vi "引用測試5.vi"() -> ()   [LabVIEW 2015]
uses:
  <vilib>/userdefined/High Color/IMAQdx.ctl
  <vilib>/vision/Measure.llb/Edge Options.ctl
  <vilib>/vision/Measure.llb/Edge Polarity.ctl
  <vilib>/vision/driver/NI_Vision_Acquisition_Software.lvlib
  <vilib>/vision/NI_Vision_Development_Module.lvlib
panel:
  out "error out 2":errorcluster
  in  "Options":T3={"Search Direction"=0, "Edge Options"={"Edge Polarity"=0, "Kernel Size"=3, "Width"=3, "Minimum Edge Strength"=10.0, "Interpolation Type"=enum."Bilinear Fixed", "Data Processing Method"=enum."Average"}, "Show Search Area"=FALSE, "Show Search Lines"=FALSE, "Show Edges Found"=FALSE, "Show Result"=TRUE, "Search Area Color"=65280, "Search Lines Color"=255, "Edge Locations Color"=16776960, "Result Color"=16711680, "Overlay Group Name"=""} {"Edge Options"."Edge Polarity" items=["All Edges", "Rising Edges", "Falling Edges"]; "Edge Options"."Minimum Edge Strength" format="%.2f"; "Edge Options"."Width" step=2; "Edge Options"."Kernel Size" step=2; "Search Direction" items=["Left to Right", "Right to Left", "Top to Bottom", "Bottom to Top"]}
  in  "Tab Control":T4(tab)
  in  "邊":T5(ring)
  out "Line Data":cluster{"X":sgl, "Y":sgl, "T":sgl}
  in  "圓":enum16{"Inner to Outer", "Outer to Inner"}(ring)
  out "Ellipse":T6 {"Minor Axis"."Point 2"."Y" format="%.2f"; "Minor Axis"."Point 2"."X" format="%.2f"; "Minor Axis"."Point 1"."Y" format="%.2f"; "Minor Axis"."Point 1"."X" format="%.2f"; "Major Axis"."Point 2"."Y" format="%.2f"; "Major Axis"."Point 2"."X" format="%.2f"; "Major Axis"."Point 1"."Y" format="%.2f"; "Major Axis"."Point 1"."X" format="%.2f"; "Center"."Y" format="%.2f"; "Center"."X" format="%.2f"}
  in  "線":enum16{"Start to End", "End to Start"}(ring)
  out "Location (Pixel)":cluster{"X":sgl, "Y":sgl}
  in  "DieArea":i32=100 min=10
  in  "ShowData":bool
  in  "抓寬度(方向)":T7(ring)=enum."Horizon(Outer to Inner)"
  in  "Settings":T8={"Contrast"=40, "Filter width"=4, "Steepness"=2, "Subsampling Ratio"=5, "Show Search Area"=FALSE, "Show Search Lines"=FALSE, "Show Edges Found"=FALSE, "Show Result"=TRUE}
  out "Distance":sgl
  in  "繪圖":bool
  in  "繪圖ROI資料":T9=enum."Set Data"
  out "Line Profile":T10(graph)
  in  "Session In":T11="cam1"
  in  "Numeric":i32
  in  "重新開圖":bool
  in  "開圖":bool
  in  "動作":enum16{"什麼也不做", "抓邊", "看灰階", "分析光源均勻度", "抓寬度"}(ring)
  out "Mean":sgl format="%#.2f"
  out "Histogram":T12(graph)
  in  "取像":bool
  out "error out":errorcluster
  out "Gradient Information":dbl[][](graph)
  in  "Process":T13(ring)
  in  "Gap":i32=10 min=1 max=300
  in  "stop":bool
  out "Image":T14(plugin-control)
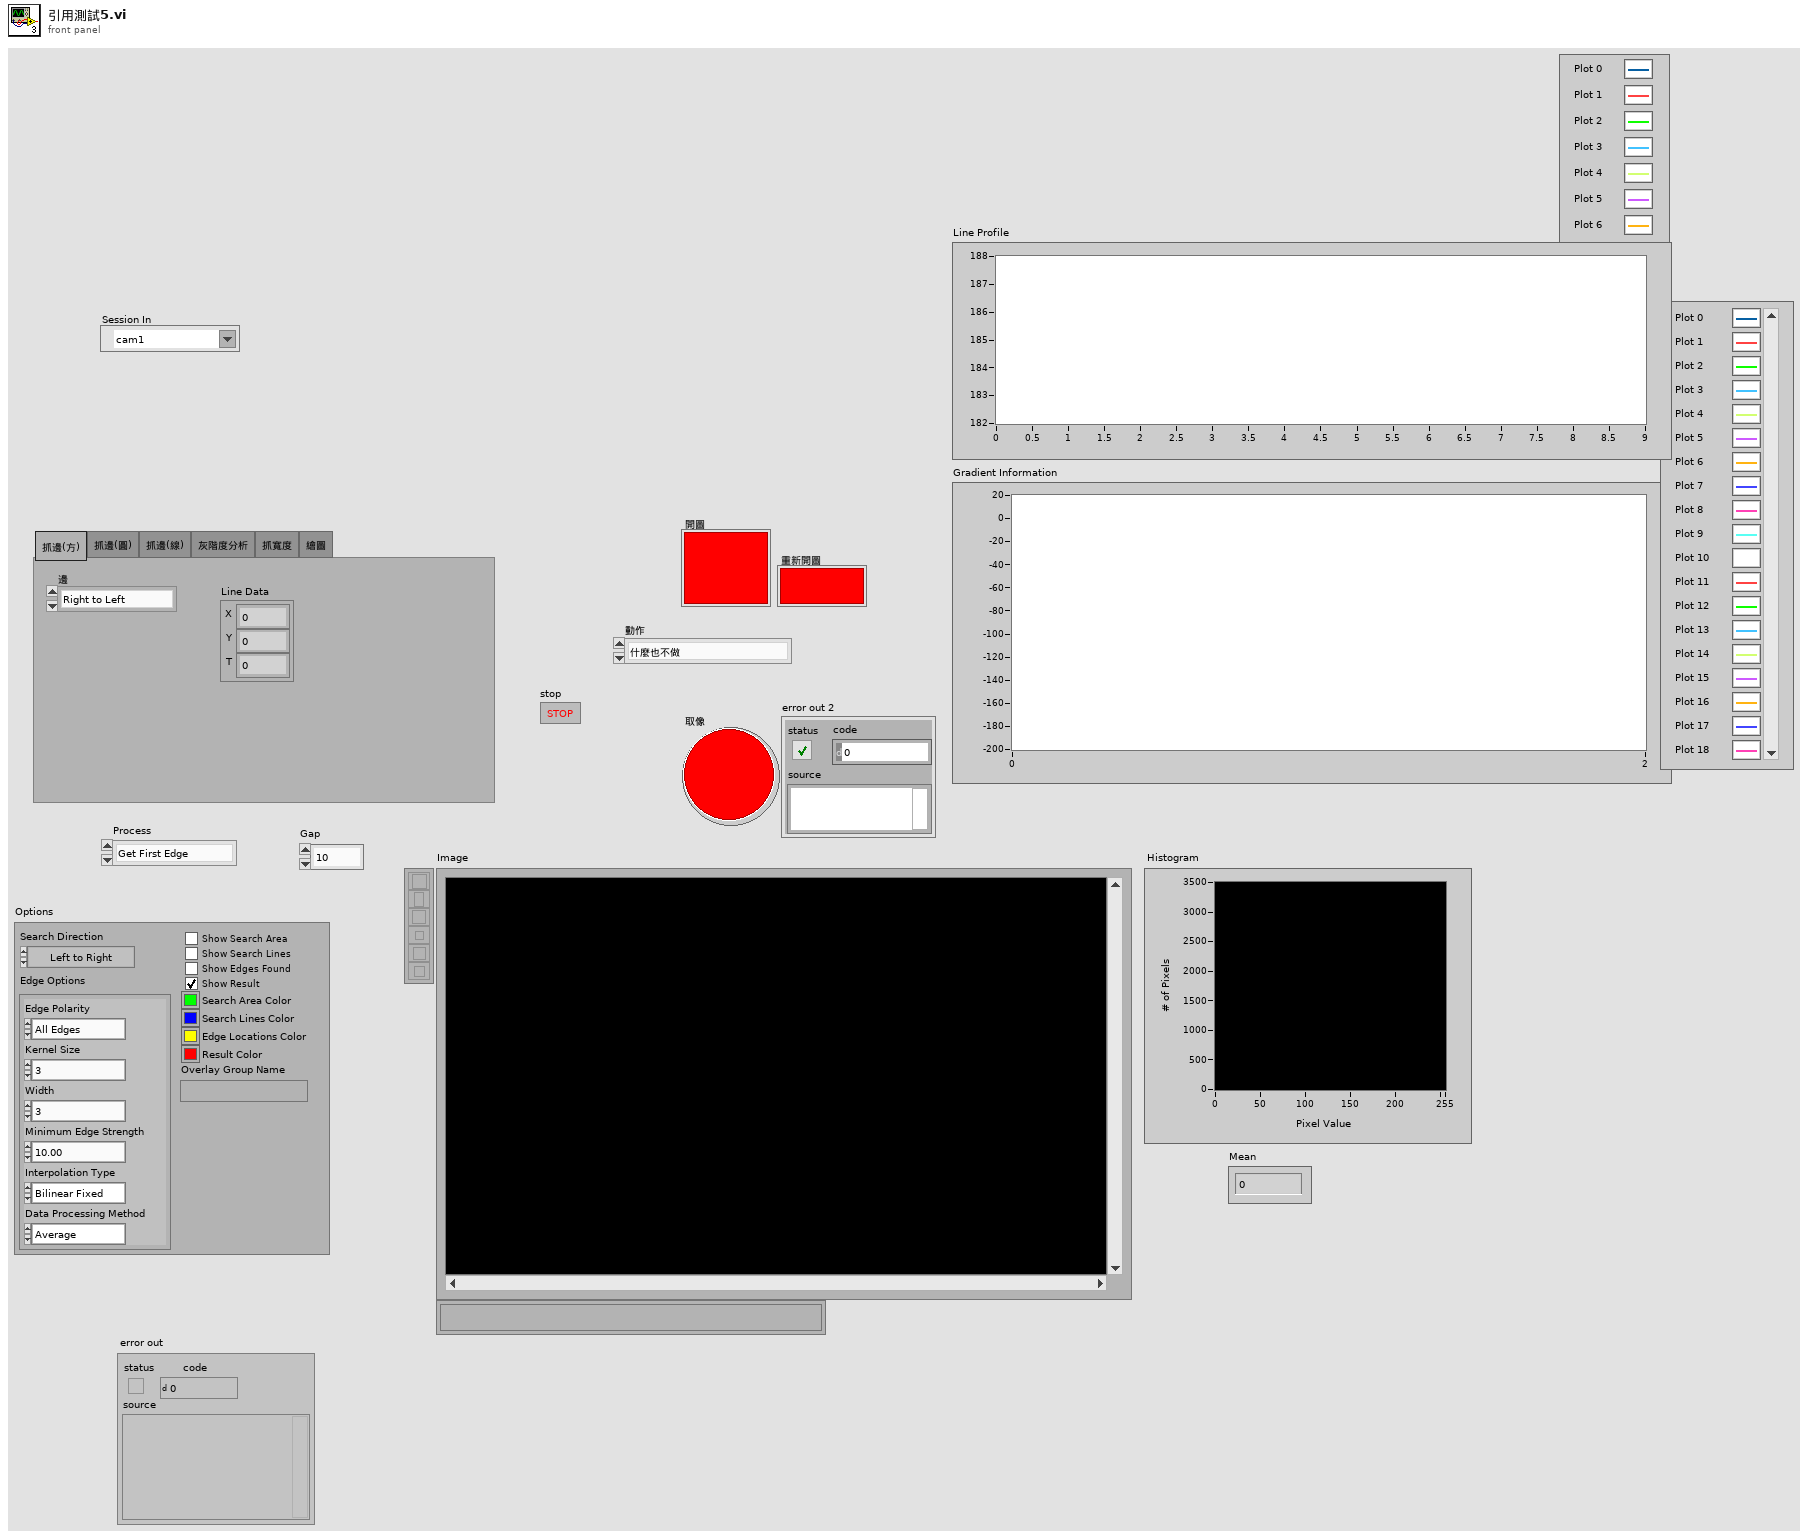
[diagram p1: front panel]
types:
  T1 = typedef "Edge Options.ctl" = cluster{"Edge Polarity":T2, "Kernel Size":u32, "Width":u32, "Minimum Edge Strength":sgl, "Interpolation Type":enum32{"Zero Order", "Bilinear", "Quadratic", "Cubic", "Bilinear Fixed"}, "Data Processing Method":enum32{"Average", "Median"}}
  T2 = typedef "Edge Polarity.ctl" = u32
  T3 = cluster{"Search Direction":u32, "Edge Options":T1, "Show Search Area":bool, "Show Search Lines":bool, "Show Edges Found":bool, "Show Result":bool, "Search Area Color":u32, "Search Lines Color":u32, "Edge Locations Color":u32, "Result Color":u32, "Overlay Group Name":string}
  T4 = enum32{"抓邊(方)", "抓邊(圓)", "抓邊(線)", "灰階度分析", "抓寬度", "繪圖"}
  T5 = enum16{"Right to Left", "Left  to Right", "Up to Down", "Down to Up"}
  T6 = cluster{"Center":cluster{"X":sgl, "Y":sgl}, "Major Axis":cluster{"Point 1":cluster{"X":sgl, "Y":sgl}, "Point 2":cluster{"X":sgl, "Y":sgl}}, "Minor Axis":cluster{"Point 1":cluster{"X":sgl, "Y":sgl}, "Point 2":cluster{"X":sgl, "Y":sgl}}}
  T7 = enum16{"Horizon(Inner to Outer)", "Horizon(Outer to Inner)", "Vertical (Inner to Outer)", "Vertical(Outer to Inner)"}
  T8 = cluster{"Contrast":i32, "Filter width":i32, "Steepness":i32, "Subsampling Ratio":u32, "Show Search Area":bool, "Show Search Lines":bool, "Show Edges Found":bool, "Show Result":bool}
  T9 = typedef "Action_Data.ctl" = enum16{"Initialize", "Get Data", "Set Data", "Delete Data", "Idle"}
  T10 = cluster{"x0":sgl, "dx":sgl, "Pixels Line":sgl[]}[]
  T11 = typedef "IMAQdx.ctl" = refnum<k21>
  T12 = cluster{"Starting Value":sgl, "Incremental Value":sgl, "Histogram":u32[]}
  T13 = enum16{"Get First Edge", "Get First + Last Edge", "Get All Edges", "Get Best Edge"}
  T14 = typedef "IMAQ Image.ctl" = refnum<image>
  T15 = typedef "IMAQ Rectangle" = cluster{"Left":i32, "Top":i32, "Right":i32, "Bottom":i32, "Rotation":dbl}
  T16 = typedef "ROI Descriptor" = cluster{"Global Rectangle":i32[], "Contours":cluster{"ID":enum32{"External", "Internal"}, "Type":u32, "Coordinates":i32[]}[]}
  T17 = cluster{"Origin":cluster{"X":sgl, "Y":sgl}, "Angle (deg)":sgl, "Axis Reference":u32}
  T18 = typedef "Image Type" = u32
  T19 = cluster{"Global Rectangle":i32[], "Contours":cluster{"Contour Type":u32, "ROI Type":u32, "Points":i32[]}[]}
  T20 = cluster{"Contour Type":u32, "ROI Type":u32, "Points":i32[]}[]
  T21 = cluster{"Contour Type":u32, "ROI Type":u32, "Points":i32[]}
  T22 = enum32{"Zero Order", "Bilinear", "Quadratic", "Cubic", "Bilinear Fixed"}
  T23 = cluster{"邊":enum16{"Right to Left", "Left  to Right", "Up to Down", "Down to Up"}, "動作":enum16{"什麼也不做", "抓邊", "看灰階", "分析光源均勻度", "抓寬度"}, "圓":enum16{"Inner to Outer", "Outer to Inner"}, "Process":enum16{"Get First Edge", "Get First + Last Edge", "Get All Edges", "Get Best Edge"}, "Gap":i32, bool, "Search Direction":u32, "Edge Polarity":T2, "Kernel Size":u32, "Width":u32, "Minimum Edge Strength":sgl, "Data Processing Method":enum32{"Average", "Median"}, "Interpolation Type":enum32{"Zero Order", "Bilinear", "Quadratic", "Cubic", "Bilinear Fixed"}, "Show Search Area":bool, "Show Search Lines":bool, "Show Edges Found":bool, "Show Result":bool, "Search Area Color":u32, "Search Lines Color":u32, "Edge Locations Color":u32, "Result Color":u32, "Overlay Group Name":string, "DieArea":i32, "ShowData":bool, "線":enum16{"Start to End", "End to Start"}, "抓寬度(方向)":enum16{"Horizon(Inner to Outer)", "Horizon(Outer to Inner)", "Vertical (Inner to Outer)", "Vertical(Outer to Inner)"}, "Contrast":i32, "Filter width":i32, "Steepness":i32, "Subsampling Ratio":u32, "Show Search Area":bool, "Show Search Lines":bool, "Show Edges Found":bool, "Show Result":bool, bool}
  T24 = cluster{"邊":bool, "動作":bool, "圓":bool, "Process":bool, "Gap":bool, bool, "Search Direction":bool, "Edge Polarity":bool, "Kernel Size":bool, "Width":bool, "Minimum Edge Strength":bool, "Data Processing Method":bool, "Interpolation Type":bool, "Show Search Area":bool, "Show Search Lines":bool, "Show Edges Found":bool, "Show Result":bool, "Search Area Color":bool, "Search Lines Color":bool, "Edge Locations Color":bool, "Result Color":bool, "Overlay Group Name":bool, "DieArea":bool, "ShowData":bool, "線":bool, "抓寬度(方向)":bool, "Contrast":bool, "Filter width":bool, "Steepness":bool, "Subsampling Ratio":bool, "Show Search Area":bool, "Show Search Lines":bool, "Show Edges Found":bool, "Show Result":bool, bool}
  T25 = cluster{"Base Reference":cluster{"Origin":cluster{"X":sgl, "Y":sgl}, "Angle (deg)":sgl, "Axis Reference":u32}, "Base Reference":cluster{"Origin":cluster{"X":sgl, "Y":sgl}, "Angle (deg)":sgl, "Axis Reference":u32}}
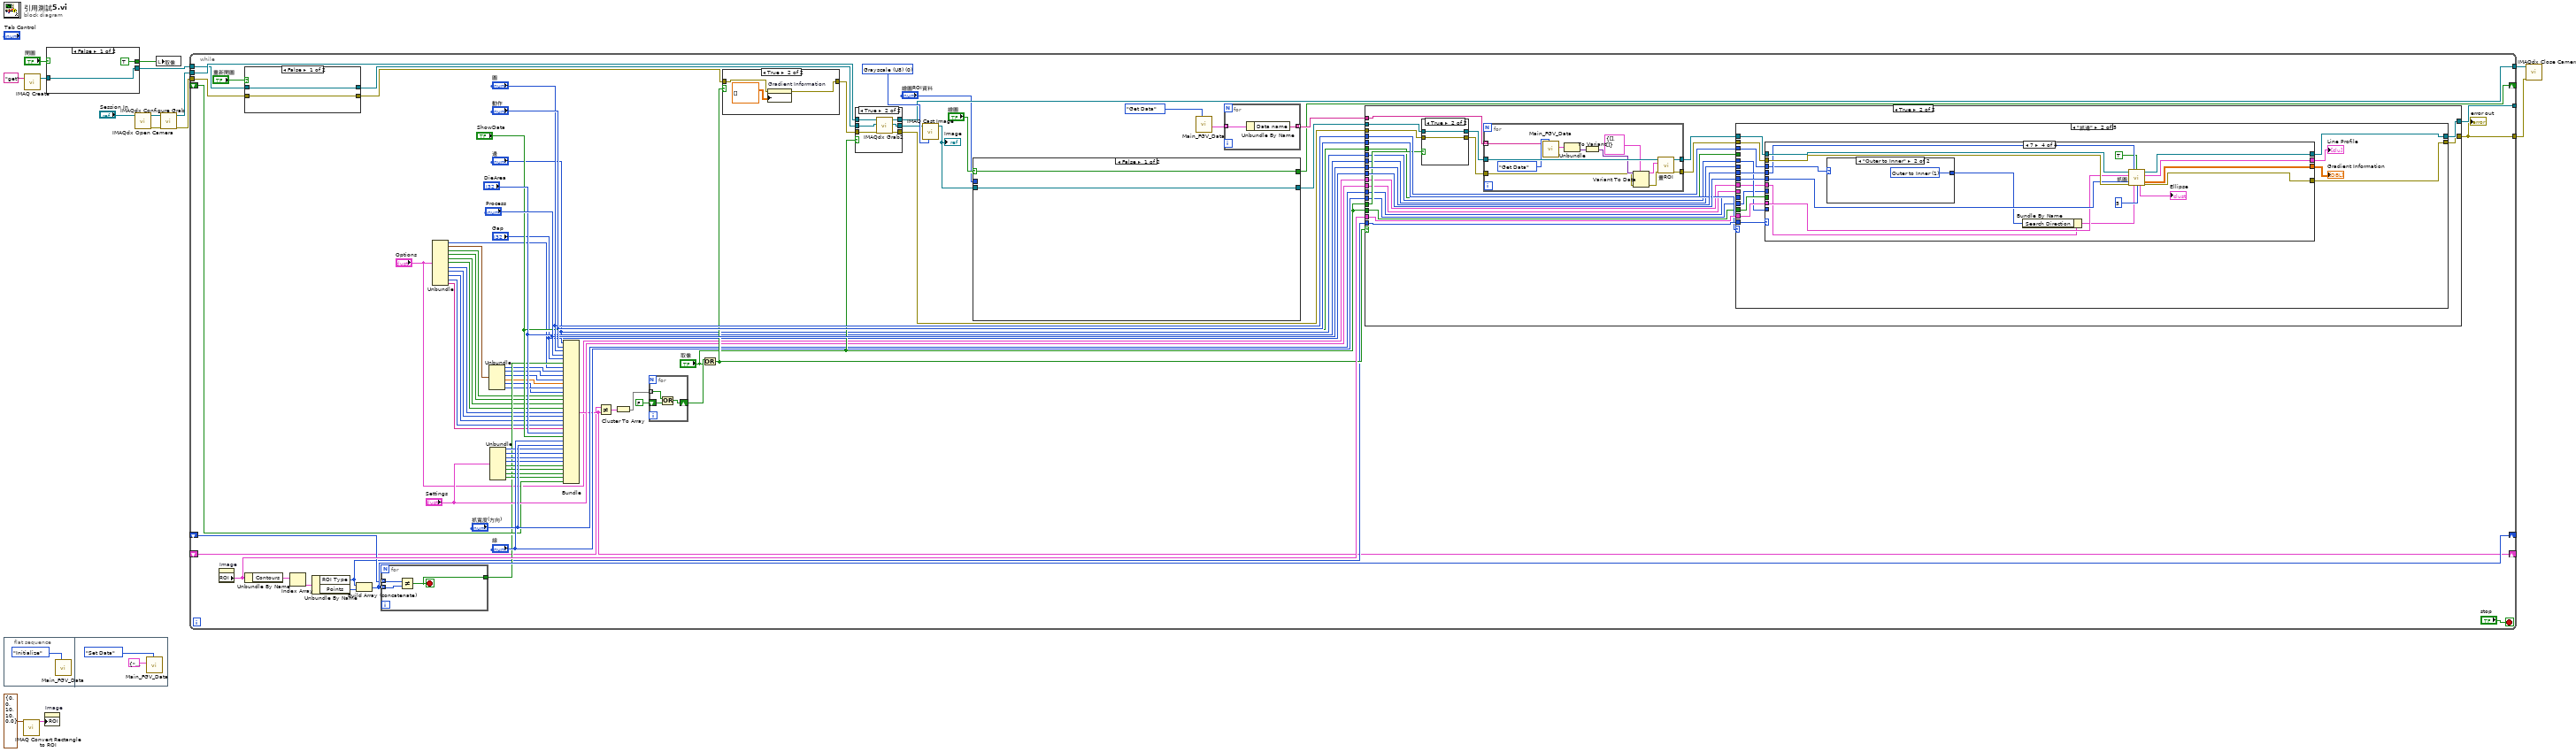
[diagram p0: block diagram]
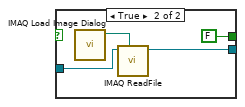
[diagram p2: hidden frame]
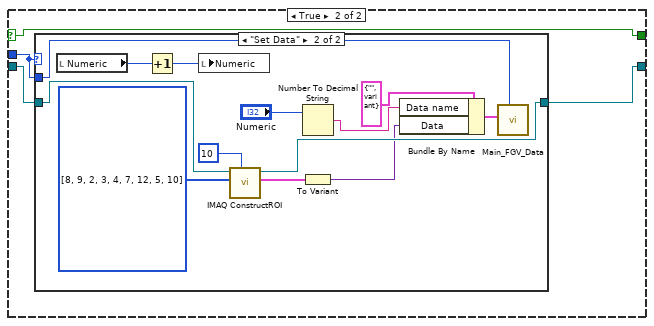
[diagram p3: hidden frame]
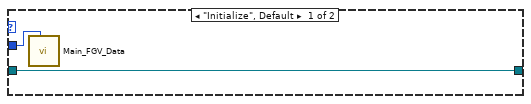
[diagram p4: hidden frame]
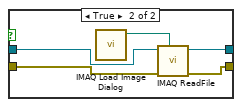
[diagram p5: hidden frame]
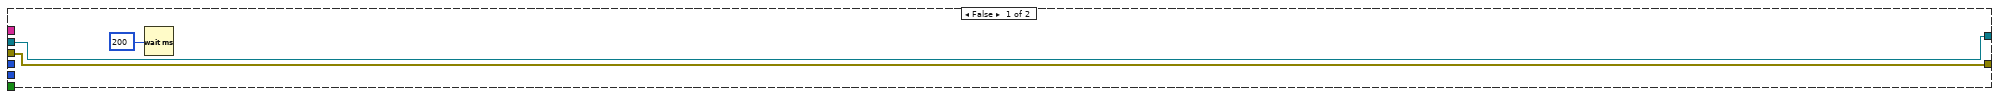
[diagram p7: hidden frame]
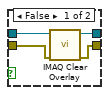
[diagram p8: hidden frame]
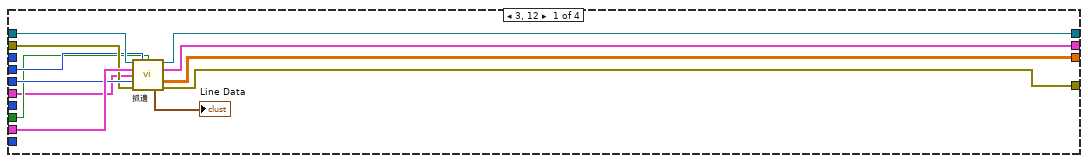
[diagram p10: hidden frame]
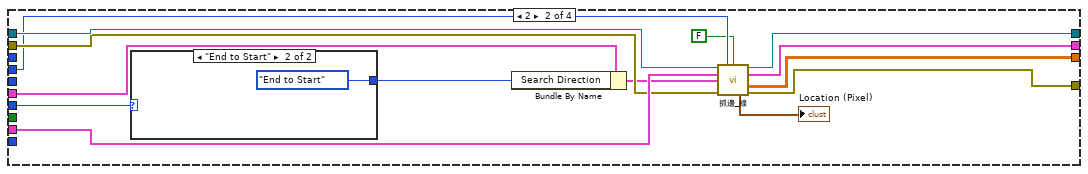
[diagram p11: hidden frame]
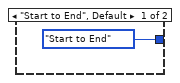
[diagram p12: hidden frame]
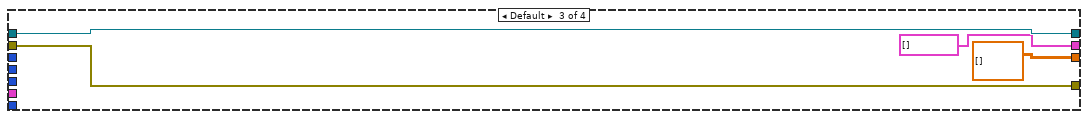
[diagram p13: hidden frame]
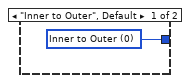
[diagram p14: hidden frame]
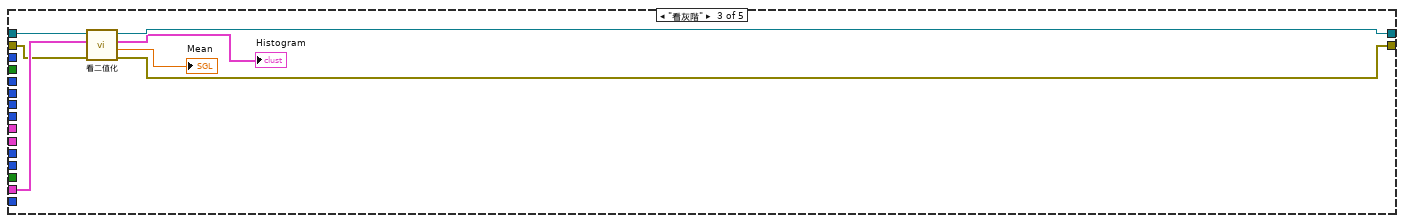
[diagram p15: hidden frame]
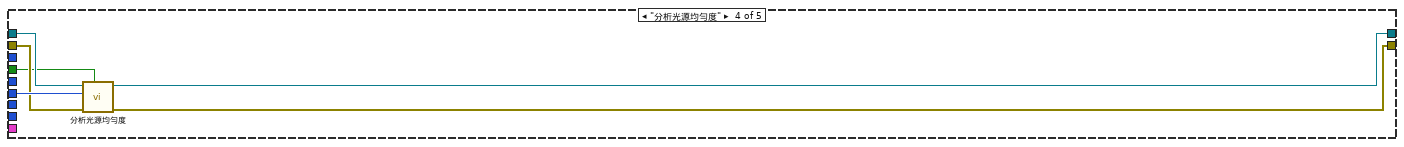
[diagram p16: hidden frame]
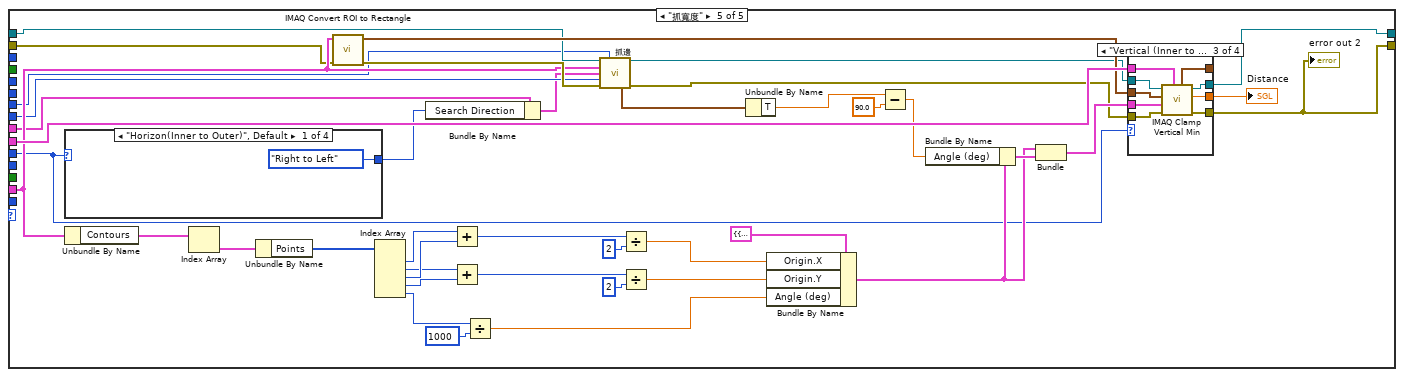
[diagram p17: hidden frame]
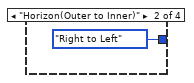
[diagram p18: hidden frame]
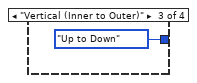
[diagram p19: hidden frame]
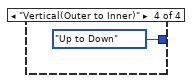
[diagram p20: hidden frame]
diagram:
  n1 = flat-sequence {
    frame #0 {
      n2 = call "Main_FGV_Data.vi"("Action_Data"=Action_Data."Initialize") -> ()  [unwired: 9 in, 2 out]
    }
    frame #1 {
      n3 = call "Main_FGV_Data.vi"("Action_Data"=Action_Data."Set Data", "Data In"=cluster{"Data name":string, "Data":variant} {"Data name"="Oringal", "Data"=variant(cluster{"Global Rectangle":i32[], "Contours":cluster{"ID":enum32{"External", "Internal"}, "Type":u32, "Coordinates":i32[]}[]} {"Global Rectangle"=[0, 959, 2, 960], "Contours"=[{"ID"=enum."External", "Type"=2, "Coordinates"=[0, 959, 1, 959]}]})} ("output cluster 3")) -> ()  [unwired: 8 in, 2 out]
    }
  }
  n4 = call "IMAQ Convert Rectangle to ROI"("Rectangle"=T15 {"Left"=0, "Top"=0, "Right"=10, "Bottom"=10, "Rotation"=0.0}) -> ("ROI Descriptor"=w7:T16)  [unwired: 8 in, 1 out]
  n5 = call "IMAQ Create"("Image Name"="get") -> ("New Image"=w4:T14)  [unwired: 4 in, 1 out]
  n6 = property on="Image" class="ImageControl"("ROI"=w7) -> ()  [unwired: 2 in, 2 out]
  n7 = case shown="False" "開圖" {
    tunnel: [TRUE ("取像") FALSE ("取像")] -> w5
    tunnel: w4 -> [w18 w22]
    tunnel: [w18 w21] -> w3
    frame False {
    }
    frame True {
      n8 = call "IMAQ Load Image Dialog"() -> ("Path"=w20:path)  [unwired: 9 in, 2 out]
      n9 = call "IMAQ ReadFile"("File Path"=w20, "Image"=w22) -> ("Image Out"=w21:T14)  [unwired: 5 in, 4 out]
    }
  }
  n10 = call <vilib>:"IMAQdx Open Camera.vi"("Session In"="Session In") -> ("error out"=w9:errorcluster, "Session Out"=w10:T11)  [unwired: 9 in]
  n11 = local write "取像"(w5) -> ()
  n12 = call <vilib>:"IMAQdx Configure Grab.vi"("error in"=w9, "Session In"=w10) -> ("error out"=w2:errorcluster, "Session Out"=w13:T11)  [unwired: 8 in]
  n13 = while {
    tunnel: w13 -> [w98]
    tunnel: w3 -> [w76]
    tunnel: [w85] -> w12
    tunnel: [w94] -> _
    tunnel: w2 -> [w65]
    tunnel: [w53] -> w1
    shift-right: [w52] -> _
    shift-left: _ -> [w51]
    shift-right: [w49] -> _
    shift-left: _ -> [w48]
    shift-right: [w44] -> _
    shift-left: _ -> [w43]
    stop <- "stop" stop-if-true
    w96 = T18 0 items=["Grayscale (U8)", "Grayscale (I16)", "Grayscale (SGL)", "Complex (CSG)", "RGB (U32)", "HSL (U32)", "RGB (U64)", "Grayscale (U16)"] ("Image Type")
    n14 = property on="Image" class="ImageControl"() -> ("ROI"=w83:T19)  [unwired: 2 in, 2 out]
    n15 = case shown="False" "重新開圖" {
      tunnel: w76 -> [w126 w129]
      tunnel: [w126 w130] -> w75
      tunnel: w65 -> [w125 w128]
      tunnel: [w125 w127] -> w64
      frame False {
      }
      frame True {
        n16 = call "IMAQ Load Image Dialog"() -> ("Path"=w131:path)  [unwired: 9 in, 2 out]
        n17 = call "IMAQ ReadFile"("File Path"=w131, "error in (no error)"=w128, "Image"=w129) -> ("error out"=w127:errorcluster, "Image Out"=w130:T14)  [unwired: 4 in, 3 out]
      }
    }
    n18 = Unbundle By Name(w83) -> ("Contours"=w93:T20)
    n19 = Index Array(array=w93) -> (element=w92:T21)  [unwired: 1 in]
    n20 = Unbundle By Name(w92) -> ("ROI Type"=w46:u32, "Points"=w50:i32[])
    n21 = Build Array (concatenate)(w46, w50) -> (w49:u32[])
    n22 = for {
      tunnel: w48 -> [w101] mode=indexing
      tunnel: w49 -> [w100] mode=indexing
      tunnel: [w99] -> w47
      stop <- w99 stop-if-true
      n23 = Not Equal?(x=w101, y=w100) -> (x != y?=w99:bool)
    }
    n24 = Unbundle("Options") -> ("Search Direction"=w41:u32, "Edge Options"=w31:T1, "Show Search Area"=w40:bool, "Show Search Lines"=w39:bool, "Show Edges Found"=w38:bool, "Show Result"=w37:bool, "Search Area Color"=w36:u32, "Search Lines Color"=w35:u32, "Edge Locations Color"=w34:u32, "Result Color"=w33:u32, "Overlay Group Name"=w32:string)
    n25 = Unbundle(w31) -> ("Edge Polarity"=w30:T2, "Kernel Size"=w29:u32, "Width"=w28:u32, "Minimum Edge Strength"=w26:sgl, "Interpolation Type"=w25:T22, "Data Processing Method"=w27:enum32{"Average", "Median"})
    n26 = Unbundle("Settings") -> ("Contrast"=w62:i32, "Filter width"=w61:i32, "Steepness"=w60:i32, "Subsampling Ratio"=w59:u32, "Show Search Area"=w58:bool, "Show Search Lines"=w57:bool, "Show Edges Found"=w56:bool, "Show Result"=w55:bool)
    n27 = Bundle("邊"="邊", "動作"="動作", "圓"="圓", "Process"="Process", "Gap"="Gap", w47, "Search Direction"=w41, "Edge Polarity"=w30, "Kernel Size"=w29, "Width"=w28, "Minimum Edge Strength"=w26, "Data Processing Method"=w27, "Interpolation Type"=w25, "Show Search Area"=w40, "Show Search Lines"=w39, "Show Edges Found"=w38, "Show Result"=w37, "Search Area Color"=w36, "Search Lines Color"=w35, "Edge Locations Color"=w34, "Result Color"=w33, "Overlay Group Name"=w32, "DieArea"="DieArea", "ShowData"="ShowData", "線"="線", "抓寬度(方向)"="抓寬度(方向)", "Contrast"=w62, "Filter width"=w61, "Steepness"=w60, "Subsampling Ratio"=w59, "Show Search Area"=w58, "Show Search Lines"=w57, "Show Edges Found"=w56, "Show Result"=w55, w51) -> (w44:T23)  [unwired: 1 in]
    n28 = Not Equal?(x=w43, y=w44) -> (x != y?=w24:T24)
    n29 = Cluster To Array(cluster=w24) -> (array=w89:bool[])
    n30 = for {
      tunnel: w89 -> [w136] mode=indexing
      shift-right: [w138] -> w87
      shift-left: FALSE -> [w137]
      n31 = Or(x=w136, y=w137) -> (x .or. y?=w138:bool)
    }
    n32 = Or(x=w87, y="取像") -> (x .or. y?=w82:bool)
    n33 = case shown="True" w82 {
      tunnel: [w132 w134] -> w95
      tunnel: w64 -> [w132 w133]
      frame False {
      }
      frame True {
        n34 = property on="Gradient Information" class="WFChart (strict)"(error in=w133, "History Data"=dbl[][] []) -> (error out=w134:errorcluster)  [unwired: 1 in, 1 out]
      }
    }
    n35 = case shown="True" "取像" {
      tunnel: w98 -> [w347 w353]
      tunnel: w75 -> [w346 w352]
      tunnel: [w347 w351] -> w85
      tunnel: [w346 w350] -> w84
      tunnel: w95 -> [w345 w349]
      tunnel: [w345 w348] -> w69
      frame False {
      }
      frame True {
        n36 = call <vilib>:"IMAQdx Grab2.vi"("error in"=w349, "Image In"=w352, "Session In"=w353) -> ("error out"=w348:errorcluster, "Image Out"=w350:T14, "Session Out"=w351:T11)  [unwired: 5 in, 1 out]
      }
    }
    n37 = call "IMAQ Cast Image"("Image Type"=w96, "Image Src"=w84) -> ("Image Dst Out"=w68:T14)  [unwired: 8 in, 1 out]
    "Image" <- w68
    n38 = case shown="False" "繪圖" {
      selector: "繪圖" -> [w104 w106]
      tunnel: w68 -> [w105 w109]
      tunnel: [w105 w108] -> w67
      tunnel: "繪圖ROI資料" -> [_ w107]
      tunnel: [w104 w106] -> w52
      frame False {
      }
      frame True {
        n39 = case shown="\"Set Data\"" w107 {
          tunnel: w109 -> [w111 w122]
          tunnel: [w111 w120] -> w108
          tunnel: w107 -> [w110 w114]
          frame "Initialize", Default {
            n40 = call "Main_FGV_Data.vi"("Action_Data"=w110) -> ()  [unwired: 9 in, 2 out]
          }
          frame "Set Data" {
            w124 = u32[] [8, 9, 2, 3, 4, 7, 12, 5, 10] items=["No Selection", "Point", "Line", "Rectangle", "Oval", "Polygon", "Freehand Region", "Annulus", "Zoom", "Pan", "Broken Line", "Freehand Line", "Rotated Rectangle"] ("Tools")
            n41 = local read "Numeric"() -> (w116:i32)
            n42 = Increment(x=w116) -> (x+1=w115:i32)
            n43 = local write "Numeric"(w115) -> ()
            n44 = call "IMAQ ConstructROI"("Window Number (-1...15)"=10, "Tools"=w124, "Image"=w122) -> ("ROI Descriptor Out"=w121:T16, "Image Out (duplicate)"=w120:T14)  [unwired: 5 in, 2 out]
            n45 = Number To Decimal String(number="Numeric") -> (decimal integer string=w113:string)  [unwired: 1 in]
            n46 = To Variant(anything=w121) -> (Variant=w119:variant)
            n47 = Bundle By Name(cluster=cluster{"Data name":string, "Data":variant} {"Data name"="", "Data"=variant} ("Data In"), "Data name"=w113, "Data"=w119) -> (w112:cluster{"Data name":string, "Data":variant})
            n48 = call "Main_FGV_Data.vi"("Action_Data"=w114, "Data In"=w112) -> ()  [unwired: 8 in, 2 out]
          }
        }
      }
    }
    n49 = call "Main_FGV_Data.vi"("Action_Data"=Action_Data."Get Data") -> ("Data Array out"=w73:cluster{"Data name":string, "Data":variant}[])  [unwired: 9 in, 1 out]
    n50 = for {
      tunnel: [w103] -> w70 mode=indexing
      tunnel: w73 -> [w102] mode=indexing
      n51 = Unbundle By Name(w102) -> ("Data name"=w103:string)
    }
    n52 = case shown="True" w82 {
      tunnel: "Gap" -> [_ w165]
      tunnel: w69 -> [w141 w151]
      tunnel: "Process" -> [_ w164]
      tunnel: w67 -> [w140 w156]
      tunnel: [w140 w163] -> w94
      tunnel: w83 -> [_ w162]
      tunnel: w46 -> [_ w161]
      tunnel: [w141 w160] -> w53
      tunnel: "動作" -> [_ w159]
      tunnel: "圓" -> [_ w158]
      tunnel: "取像" -> [_ w157]
      tunnel: "取像" -> [_ w155]
      tunnel: "DieArea" -> [_ w154]
      tunnel: "ShowData" -> [_ w153]
      tunnel: "邊" -> [_ w152]
      tunnel: w70 -> [_ w149]
      tunnel: "線" -> [_ w145]
      tunnel: "抓寬度(方向)" -> [_ w144]
      tunnel: "Settings" -> [_ w143]
      tunnel: "Options" -> [_ w142]
      frame False {
        n53 = Wait (ms)(milliseconds to wait=u32 200) -> ()  [unwired: 1 out]
      }
      frame True {
        n54 = case shown="True" w157 {
          tunnel: w156 -> [w180 w183]
          tunnel: [w181 w183] -> w147
          tunnel: w151 -> [w179 w182]
          tunnel: [w178 w182] -> w148
          frame False {
            n55 = call "IMAQ Clear Overlay"("error in (no error)"=w179, "Image"=w180) -> ("error out"=w178:errorcluster, "Image Out"=w181:T14)  [unwired: 8 in]
          }
          frame True {
          }
        }
        n56 = for {
          tunnel: w147 -> [w177]
          tunnel: [w176] -> w146
          tunnel: w148 -> [w167]
          tunnel: [w166] -> w150
          tunnel: w149 -> [w168] mode=indexing
          n57 = call "Main_FGV_Data.vi"("Action_Data"=Action_Data."Get Data", "Data name"=w168) -> ("Data  Out"=w174:cluster{"Data name":string, "Data":variant})  [unwired: 8 in, 1 out]
          n58 = Unbundle(w174) -> ("Data"=w173:variant)  [unwired: 1 out]
          n59 = To Variant(anything=w173) -> (Variant=w172:variant)
          n60 = Variant To Data(error in=w167, type=T16 {"Global Rectangle"=[], "Contours"=[]} ("ROI Descriptor"), Variant=w172) -> (data=w170:T16, error out=w169:errorcluster)
          n61 = call "畫ROI.vi"("error in (no error)"=w169, "ROI In"=w170, "Image In"=w177) -> ("error out"=w166:errorcluster, "Image Out"=w176:T14)  [unwired: 7 in]
        }
        n62 = case shown="\"抓邊\"" w159 {
          tunnel: w165 -> [_ w200 _ _ w268]
          tunnel: w150 -> [w184 w189 w254 w259 w274]
          tunnel: w158 -> [_ w199 _ _ _]
          tunnel: w164 -> [_ w198 _ _ w269]
          tunnel: w146 -> [w185 w197 w256 w261 w271]
          tunnel: [w185 w196 w257 w262 w304] -> w163
          tunnel: w162 -> [_ w195 w255 _ w275]
          tunnel: w161 -> [_ w194 _ _ _]
          tunnel: [w184 w192 w251 w263 w302] -> w160
          tunnel: w155 -> [_ w191 _ _ _]
          tunnel: w154 -> [_ _ _ w260 _]
          tunnel: w153 -> [_ _ _ w258 _]
          tunnel: w152 -> [_ w190 _ _ _]
          tunnel: w145 -> [_ w188 _ _ _]
          tunnel: w144 -> [_ _ _ _ w272]
          tunnel: w143 -> [_ _ _ _ w301]
          tunnel: w142 -> [_ w186 _ _ w266]
          frame "什麼也不做", Default {
          }
          frame "抓邊" {
            n63 = case shown="7" w194 {
              tunnel: w195 -> [w211 w226 _ w245]
              tunnel: w200 -> [w210 _ _ w246]
              tunnel: w189 -> [w209 w224 w230 w247]
              tunnel: w199 -> [_ _ _ w236]
              tunnel: w198 -> [w205 w221 _ w243]
              tunnel: [w207 w220 dbl[][] [] ("Gradient Information") w248] -> w193
              tunnel: w197 -> [w212 w225 w232 w244]
              tunnel: [w206 w222 w232 w239] -> w196
              tunnel: [w208 w223 w230 w241] -> w192
              tunnel: w191 -> [w204 _ _ _]
              tunnel: w190 -> [_ _ _ _]
              tunnel: w188 -> [_ w216 _ _]
              tunnel: [w202 w218 T10 [] ("Line Profile") w237] -> w187
              tunnel: w186 -> [w201 w213 _ w235]
              frame 3, 12 {
                n64 = call "抓邊.vi"("Image In"=w212, "Process"=w205, "Optimized Mode"=w204, "ROI"=w211, "Options"=w201, "Gap"=w210, "error In"=w209) -> ("Image Out"=w206:T14, "Line Profile"=w202:T10, "Gradient Information"=w207:dbl[][], "Line Data"=→"Line Data":cluster{"X":sgl, "Y":sgl, "T":sgl}, "error out"=w208:errorcluster)  [unwired: 3 in, 1 out]
              }
              frame 2 {
                n65 = case shown="\"End to Start\"" w216 {
                  tunnel: [enum16{"Start to End", "End to Start"}."Start to End" ("Direction") enum16{"Start to End", "End to Start"}."End to Start" ("Direction")] -> w215
                  frame "Start to End", Default {
                  }
                  frame "End to Start" {
                  }
                }
                n66 = Bundle By Name(cluster=w213, "Search Direction"=w215) -> (w214:T3)
                n67 = call "抓邊_線.vi"("Image In"=w225, "Process"=w221, "Optimized Mode"=FALSE, "ROI"=w226, "Options"=w214, "error In"=w224) -> ("Image Out"=w222:T14, "Line Profile"=w218:T10, "Gradient Information"=w220:dbl[][], "Location (Pixel)"=→"Location (Pixel)":cluster{"X":sgl, "Y":sgl}, "error out"=w223:errorcluster)  [unwired: 5 in]
              }
              frame Default {
              }
              frame 7 {
                n68 = case shown="\"Outer to Inner\"" w236 {
                  tunnel: [w249 w250] -> w234
                  frame "Inner to Outer", Default {
                    w249 = u32 0 items=["Inner to Outer", "Outer to Inner"] ("Search Direction")
                  }
                  frame "Outer to Inner" {
                    w250 = u32 1 items=["Inner to Outer", "Outer to Inner"] ("Search Direction")
                  }
                }
                n69 = Bundle By Name(cluster=w235, "Search Direction"=w234) -> (w233:T3)
                n70 = call "抓圓.vi"("Image In"=w244, "Process"=w243, "Optimized Mode"=TRUE, "ROI"=w245, "Gap"=w246, "error In"=w247, "Options"=w233, "Point Diameter (5)"=u32 5) -> ("Imag e Out"=w239:T14, "Line Profile"=w237:T10, "Gradient Information"=w248:dbl[][], "Ellipse"=→"Ellipse":T6, "error out"=w241:errorcluster)  [unwired: 3 in]
              }
            }
            "Gradient Information" <- w193
            "Line Profile" <- w187
          }
          frame "看灰階" {
            n71 = call "看二值化.vi"("error in (no error)"=w254, "ROI Descriptor"=w255, "Image In"=w256) -> ("error out"=w251:errorcluster, "Mean"=→"Mean":sgl, "Histogram"=→"Histogram":T12, "Image Out"=w257:T14)  [unwired: 4 in, 1 out]
          }
          frame "分析光源均勻度" {
            n72 = call "分析光源均勻度.vi"("ShowData"=w258, "error in (no error)"=w259, "DieArea"=w260, "Image In"=w261) -> ("error out"=w263:errorcluster, "Image"=w262:T14)  [unwired: 6 in]
          }
          frame "抓寬度" {
            n73 = case shown="\"Horizon(Inner to Outer)\", Default" w272 {
              tunnel: [T5."Right to Left" ("Direction") T5."Right to Left" ("Direction") T5."Up to Down" ("Direction") T5."Up to Down" ("Direction")] -> w265
              frame "Horizon(Inner to Outer)", Default {
              }
              frame "Horizon(Outer to Inner)" {
              }
              frame "Vertical (Inner to Outer)" {
              }
              frame "Vertical(Outer to Inner)" {
              }
            }
            n74 = Unbundle By Name(w275) -> ("Contours"=w296:T20)
            n75 = Index Array(array=w296) -> (element=w295:T21)  [unwired: 1 in]
            n76 = Unbundle By Name(w295) -> ("Points"=w291:i32[])
            n77 = call "IMAQ Convert ROI to Rectangle"("error in (no error)"=w274, "ROI Descriptor"=w275) -> ("error out"=w280:errorcluster, "Rectangle"=w276:T15)  [unwired: 7 in]
            n78 = Index Array(array=w291) -> (element #1=w290:i32, element #2=w288:i32, element #3=w289:i32, element #4=w287:i32, element #5=w278:i32)  [unwired: 5 in]
            n79 = Bundle By Name(cluster=w266, "Search Direction"=w265) -> (w267:T3)
            n80 = Add(x=w290, y=w289) -> (x+y=w285:i32)
            n81 = Add(x=w288, y=w287) -> (x+y=w286:i32)
            n82 = Divide(x=w278, y=1000) -> (x/y=w293:dbl)
            n83 = call "抓邊.vi"("Image In"=w271, "Process"=w269, "ROI"=w275, "Options"=w267, "Gap"=w268, "error In"=w280) -> ("Image Out"=w270:T14, "Line Data"=w264:cluster{"X":sgl, "Y":sgl, "T":sgl}, "error out"=w273:errorcluster)  [unwired: 4 in, 3 out]
            n84 = Divide(x=w285, y=2) -> (x/y=w282:dbl)
            n85 = Divide(x=w286, y=2) -> (x/y=w281:dbl)
            n86 = Unbundle By Name(w264) -> ("T"=w297:sgl)
            n87 = Bundle By Name(cluster=T17 {"Origin"={"X"=0.0, "Y"=0.0}, "Angle (deg)"=0.0, "Axis Reference"=0} ("Base Reference"), "Origin.X"=w282, "Origin.Y"=w281, "Angle (deg)"=w293) -> (w279:T17)
            n88 = Subtract(x=w297, y=sgl 90.0) -> (x-y=w292:sgl)
            n89 = Bundle By Name(cluster=w279, "Angle (deg)"=w292) -> (w299:T17)
            n90 = Bundle("Base Reference"=w279, "Base Reference"=w299) -> (w277:T25)  [unwired: 1 in]
            n91 = case shown="\"Vertical (Inner to Outer)\"" w272 {
              tunnel: w270 -> [w317 w326 w334 w342]
              tunnel: [w316 w323 w332 w341] -> w304
              tunnel: w276 -> [w315 w324 w335 w343]
              tunnel: w273 -> [w314 w325 w333 w344]
              tunnel: [w313 w322 w331 w340] -> w303
              tunnel: [w312 w321 w330 w339] -> w302
              tunnel: w301 -> [w310 w320 w329 w338]
              tunnel: [w311 w319 w328 w337] -> _
              tunnel: w277 -> [w309 w318 w327 w336]
              frame "Horizon(Inner to Outer)", Default {
                n92 = call "IMAQ Clamp Horizontal Min"("Settings"=w310, "error in (no error)"=w314, "Coordinate System"=w309, "Rectangle"=w315, "Image"=w317) -> ("error out"=w312:errorcluster, "Distance"=w313:sgl, "Image Out"=w316:T14, "Edge Coordinates"=w311:cluster{"X":sgl, "Y":sgl}[])  [unwired: 2 in, 1 out]
              }
              frame "Horizon(Outer to Inner)" {
                n93 = call "IMAQ Clamp Horizontal Max"("Settings"=w320, "error in (no error)"=w325, "Coordinate System"=w318, "Rectangle"=w324, "Image"=w326) -> ("error out"=w321:errorcluster, "Distance"=w322:sgl, "Image Out"=w323:T14, "Edge Coordinates"=w319:cluster{"X":sgl, "Y":sgl}[])  [unwired: 2 in, 1 out]
              }
              frame "Vertical (Inner to Outer)" {
                n94 = call "IMAQ Clamp Vertical Min"("Settings"=w329, "error in (no error)"=w333, "Coordinate System"=w327, "Rectangle"=w335, "Image"=w334) -> ("error out"=w330:errorcluster, "Distance"=w331:sgl, "Image Out"=w332:T14, "Edge Coordinates"=w328:cluster{"X":sgl, "Y":sgl}[])  [unwired: 2 in, 1 out]
              }
              frame "Vertical(Outer to Inner)" {
                n95 = call "IMAQ Clamp Vertical Max"("Settings"=w338, "error in (no error)"=w344, "Coordinate System"=w336, "Rectangle"=w343, "Image"=w342) -> ("error out"=w339:errorcluster, "Distance"=w340:sgl, "Image Out"=w341:T14, "Edge Coordinates"=w337:cluster{"X":sgl, "Y":sgl}[])  [unwired: 2 in, 1 out]
              }
            }
            "Distance" <- w303
            "error out 2" <- w302
          }
        }
      }
    }
    "error out" <- w53
  }
  n96 = call <vilib>:"IMAQdx Close Camera.vi"("error in"=w1, "Session In"=w12) -> ()  [unwired: 9 in, 1 out]
